vi "Test Subpanel Val.vi"(10 "valUpdate":refnum<user-event>, 11 "evtReg":refnum<event-registration>) -> ()   [LabVIEW 2014]
panel:
  in  "Val":dbl
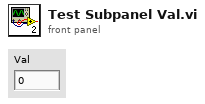
[diagram p1: front panel]
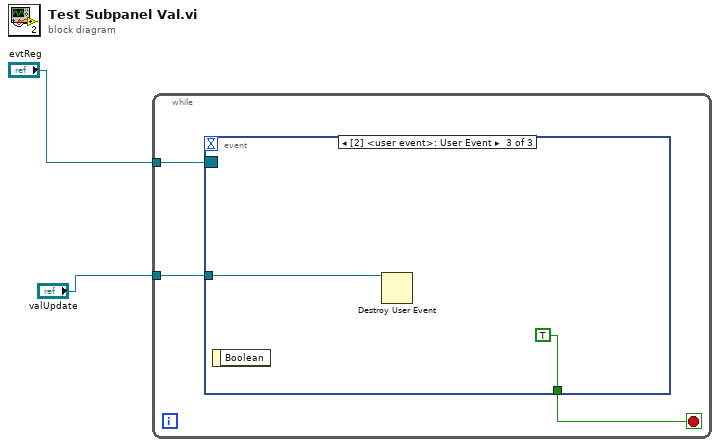
[diagram p0: block diagram]
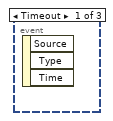
[diagram p2: hidden frame]
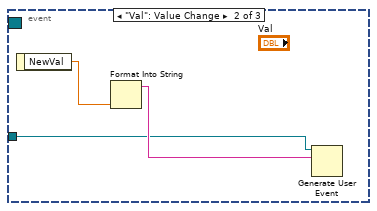
[diagram p3: hidden frame]
diagram:
  n1 = while {
    tunnel: "evtReg" -> [w5]
    tunnel: "valUpdate" -> [w3]
    stop <- w4 stop-if-true
    n2 = event shown="[2] <user event>: User Event" {
      selector: w5 -> [_ _ _]
      dyn-events: _ -> [_ _ _]
      timeout: _ -> [_ _ _]
      tunnel: [_ _ TRUE] -> w4
      tunnel: w3 -> [_ w6 w9]
      event Timeout {
        n3 = event-data() -> ()  [unwired: 1 in, 3 out]
      }
      event "Val": Value Change {
        n4 = event-data() -> ("NewVal"=w8:dbl)  [unwired: 1 in]
        n5 = Format Into String(w8) -> (resulting string=w7:string)  [unwired: 3 in, 1 out]
        n6 = Generate User Event(user event=w6, event data cluster=w7) -> ()  [unwired: 2 in, 2 out]
      }
      event User Event {
        n7 = event-data() -> ()  [unwired: 1 in, 1 out]
        n8 = Destroy User Event(user event=w9) -> ()  [unwired: 1 in, 1 out]
      }
    }
  }
